vi "Lab Panel V6.00.vi"() -> ()   [LabVIEW 2017] (continued)
                n2534 = case shown="True" w4583 {
                  tunnel: w4587 -> [_ w4592]
                  tunnel: w4586 -> [_ w4591]
                  tunnel: w4585 -> [_ w4589]
                  tunnel: w4584 -> [_ w4588]
                  frame False {
                  }
                  frame True {
                    n2535 = local read "DISP LAB04-1"() -> (w4593:T4)
                    n2536 = local read "SIG LAB04-1"() -> (w4594:T2)
                    n2537 = local read "ON L04-1"() -> (w4590:cluster{"amps":dbl, "volts":dbl, "pf":dbl})
                    n2538 = Unbundle(w4594) -> ("AMPS"=w4600:dbl, "VOLTS"=w4598:dbl, "PF"=w4597:dbl, "Tmp Live"=w4596:dbl, "Tmp Neut"=w4599:dbl)
                    n2539 = Unbundle(w4593) -> ("CYCLE"=w4595:dbl)  [unwired: 2 out]
                    n2540 = stacked-sequence {
                      tunnel: w4600 -> [w4604 w4623]
                      tunnel: w4599 -> [_ w4622]
                      tunnel: w4598 -> [w4603 w4621]
                      tunnel: w4597 -> [w4602 w4620]
                      tunnel: w4596 -> [_ w4619]
                      tunnel: w4595 -> [_ w4618]
                      tunnel: w4592 -> [_ w4617]
                      tunnel: w4591 -> [w4605 _]
                      tunnel: w4590 -> [w4601 w4615]
                      tunnel: w4589 -> [_ w4616]
                      tunnel: w4588 -> [_ w4611]
                      frame #0 {
                        n2541 = case shown="True" w4605 {
                          tunnel: w4604 -> [_ w4610]
                          tunnel: w4603 -> [_ w4609]
                          tunnel: w4602 -> [_ w4608]
                          tunnel: w4601 -> [_ w4606]
                          frame False {
                          }
                          frame True {
                            n2542 = Bundle(cluster=w4606, "amps"=w4610, "volts"=w4609, "pf"=w4608) -> (w4607:cluster{"amps":dbl, "volts":dbl, "pf":dbl})
                            n2543 = local write "ON L04-1"(w4607) -> ()
                          }
                        }
                      }
                      frame #1 {
                        n2544 = Unbundle(w4615) -> ("amps"=w4614:dbl, "volts"=w4613:dbl, "pf"=w4612:dbl)
                        n2545 = case shown="True" w4616 {
                          tunnel: w4623 -> [_ w4655]
                          tunnel: w4622 -> [_ w4662]
                          tunnel: w4621 -> [_ _]
                          tunnel: w4620 -> [_ _]
                          tunnel: w4619 -> [_ w4661]
                          tunnel: w4618 -> [_ w4660]
                          tunnel: w4617 -> [_ w4625]
                          tunnel: w4614 -> [_ w4657]
                          tunnel: w4613 -> [_ w4656]
                          tunnel: w4612 -> [_ w4654]
                          tunnel: w4611 -> [_ w4646]
                          frame False {
                          }
                          frame True {
                            n2546 = local read "TDMS LAB04-1"() -> (w4659:refnum<k34>)
                            n2547 = Build Array(w4656) -> (w4651:dbl[])
                            n2548 = Build Array(w4654) -> (w4650:dbl[])
                            n2549 = Build Array(w4661) -> (w4649:dbl[])
                            n2550 = Build Array(w4662) -> (w4648:dbl[])
                            n2551 = Build Array(w4657) -> (w4653:dbl[])
                            n2552 = Build Array(w4655) -> (w4652:dbl[])
                            n2553 = Build Array(w4660) -> (w4647:dbl[])
                            n2554 = Build Array("AMPS ON", "AMPS OFF", "VOLTS", "PF", "TEMP Live", "TEMP Neut", "CYCLE") -> (w4630:string[])
                            n2555 = Bundle By Name("Y"=w4653, "t0"=w4646) -> (w4645:waveform(dbl))  [unwired: 1 in]
                            n2556 = Bundle By Name("Y"=w4652, "t0"=w4646) -> (w4644:waveform(dbl))  [unwired: 1 in]
                            n2557 = Bundle By Name("Y"=w4651, "t0"=w4646) -> (w4643:waveform(dbl))  [unwired: 1 in]
                            n2558 = Bundle By Name("Y"=w4650, "t0"=w4646) -> (w4642:waveform(dbl))  [unwired: 1 in]
                            n2559 = Bundle By Name("Y"=w4649, "t0"=w4646) -> (w4641:waveform(dbl))  [unwired: 1 in]
                            n2560 = Bundle By Name("Y"=w4648, "t0"=w4646) -> (w4640:waveform(dbl))  [unwired: 1 in]
                            n2561 = Bundle By Name("Y"=w4647, "t0"=w4646) -> (w4639:waveform(dbl))  [unwired: 1 in]
                            n2562 = Build Array(w4645, w4644, w4643, w4642, w4641, w4640, w4639) -> (w4638:waveform(dbl)[])
                            n2563 = TDMS Write(0:w4659, 5:"TEST VALUES", 7:w4630, 9:w4638) -> (4:w4629:refnum<k34>, 6:w4628:string, 15:w4627:errorcluster)  [unwired: 2 in, 1 out]
                            n2564 = TDMS Write(0:w4629, 5:w4628, 7:"TIME", 9:w4625, 11:w4627) -> (15:w4624:errorcluster)  [unwired: 1 in, 3 out]
                            n2565 = local write "data file error"(w4624) -> ()
                          }
                        }
                      }
                    }
                  }
                }
              }
              frame #7 {
                n2566 = case shown="True" w4663 {
                  tunnel: w4667 -> [_ w4672]
                  tunnel: w4666 -> [_ w4671]
                  tunnel: w4665 -> [_ w4669]
                  tunnel: w4664 -> [_ w4668]
                  frame False {
                  }
                  frame True {
                    n2567 = local read "DISP LAB04-2"() -> (w4673:T4)
                    n2568 = local read "SIG LAB04-2"() -> (w4674:T2)
                    n2569 = local read "ON L04-2"() -> (w4670:cluster{"amps":dbl, "volts":dbl, "pf":dbl})
                    n2570 = Unbundle(w4674) -> ("AMPS"=w4680:dbl, "VOLTS"=w4678:dbl, "PF"=w4677:dbl, "Tmp Live"=w4676:dbl, "Tmp Neut"=w4679:dbl)
                    n2571 = Unbundle(w4673) -> ("CYCLE"=w4675:dbl)  [unwired: 2 out]
                    n2572 = stacked-sequence {
                      tunnel: w4680 -> [w4684 w4703]
                      tunnel: w4679 -> [_ w4702]
                      tunnel: w4678 -> [w4683 w4701]
                      tunnel: w4677 -> [w4682 w4700]
                      tunnel: w4676 -> [_ w4699]
                      tunnel: w4675 -> [_ w4698]
                      tunnel: w4672 -> [_ w4697]
                      tunnel: w4671 -> [w4685 _]
                      tunnel: w4670 -> [w4681 w4695]
                      tunnel: w4669 -> [_ w4696]
                      tunnel: w4668 -> [_ w4691]
                      frame #0 {
                        n2573 = case shown="True" w4685 {
                          tunnel: w4684 -> [_ w4690]
                          tunnel: w4683 -> [_ w4689]
                          tunnel: w4682 -> [_ w4688]
                          tunnel: w4681 -> [_ w4686]
                          frame False {
                          }
                          frame True {
                            n2574 = Bundle(cluster=w4686, "amps"=w4690, "volts"=w4689, "pf"=w4688) -> (w4687:cluster{"amps":dbl, "volts":dbl, "pf":dbl})
                            n2575 = local write "ON L04-2"(w4687) -> ()
                          }
                        }
                      }
                      frame #1 {
                        n2576 = Unbundle(w4695) -> ("amps"=w4694:dbl, "volts"=w4693:dbl, "pf"=w4692:dbl)
                        n2577 = case shown="True" w4696 {
                          tunnel: w4703 -> [_ w4735]
                          tunnel: w4702 -> [_ w4742]
                          tunnel: w4701 -> [_ _]
                          tunnel: w4700 -> [_ _]
                          tunnel: w4699 -> [_ w4741]
                          tunnel: w4698 -> [_ w4740]
                          tunnel: w4697 -> [_ w4705]
                          tunnel: w4694 -> [_ w4737]
                          tunnel: w4693 -> [_ w4736]
                          tunnel: w4692 -> [_ w4734]
                          tunnel: w4691 -> [_ w4726]
                          frame False {
                          }
                          frame True {
                            n2578 = local read "TDMS LAB04-2"() -> (w4739:refnum<k34>)
                            n2579 = Build Array(w4736) -> (w4731:dbl[])
                            n2580 = Build Array(w4734) -> (w4730:dbl[])
                            n2581 = Build Array(w4741) -> (w4729:dbl[])
                            n2582 = Build Array(w4742) -> (w4728:dbl[])
                            n2583 = Build Array(w4737) -> (w4733:dbl[])
                            n2584 = Build Array(w4735) -> (w4732:dbl[])
                            n2585 = Build Array(w4740) -> (w4727:dbl[])
                            n2586 = Build Array("AMPS ON", "AMPS OFF", "VOLTS", "PF", "TEMP Live", "TEMP Neut", "CYCLE") -> (w4710:string[])
                            n2587 = Bundle By Name("Y"=w4733, "t0"=w4726) -> (w4725:waveform(dbl))  [unwired: 1 in]
                            n2588 = Bundle By Name("Y"=w4732, "t0"=w4726) -> (w4724:waveform(dbl))  [unwired: 1 in]
                            n2589 = Bundle By Name("Y"=w4731, "t0"=w4726) -> (w4723:waveform(dbl))  [unwired: 1 in]
                            n2590 = Bundle By Name("Y"=w4730, "t0"=w4726) -> (w4722:waveform(dbl))  [unwired: 1 in]
                            n2591 = Bundle By Name("Y"=w4729, "t0"=w4726) -> (w4721:waveform(dbl))  [unwired: 1 in]
                            n2592 = Bundle By Name("Y"=w4728, "t0"=w4726) -> (w4720:waveform(dbl))  [unwired: 1 in]
                            n2593 = Bundle By Name("Y"=w4727, "t0"=w4726) -> (w4719:waveform(dbl))  [unwired: 1 in]
                            n2594 = Build Array(w4725, w4724, w4723, w4722, w4721, w4720, w4719) -> (w4718:waveform(dbl)[])
                            n2595 = TDMS Write(0:w4739, 5:"TEST VALUES", 7:w4710, 9:w4718) -> (4:w4709:refnum<k34>, 6:w4708:string, 15:w4707:errorcluster)  [unwired: 2 in, 1 out]
                            n2596 = TDMS Write(0:w4709, 5:w4708, 7:"TIME", 9:w4705, 11:w4707) -> (15:w4704:errorcluster)  [unwired: 1 in, 3 out]
                            n2597 = local write "data file error"(w4704) -> ()
                          }
                        }
                      }
                    }
                  }
                }
              }
              frame #8 {
                n2598 = case shown="True" w4743 {
                  tunnel: w4747 -> [_ w4752]
                  tunnel: w4746 -> [_ w4751]
                  tunnel: w4745 -> [_ w4749]
                  tunnel: w4744 -> [_ w4748]
                  frame False {
                  }
                  frame True {
                    n2599 = local read "DISP LAB05-1"() -> (w4753:T4)
                    n2600 = local read "SIG LAB05-1"() -> (w4754:T2)
                    n2601 = local read "ON L05-1"() -> (w4750:cluster{"amps":dbl, "volts":dbl, "pf":dbl})
                    n2602 = Unbundle(w4754) -> ("AMPS"=w4760:dbl, "VOLTS"=w4758:dbl, "PF"=w4757:dbl, "Tmp Live"=w4756:dbl, "Tmp Neut"=w4759:dbl)
                    n2603 = Unbundle(w4753) -> ("CYCLE"=w4755:dbl)  [unwired: 2 out]
                    n2604 = stacked-sequence {
                      tunnel: w4760 -> [w4764 w4783]
                      tunnel: w4759 -> [_ w4782]
                      tunnel: w4758 -> [w4763 w4781]
                      tunnel: w4757 -> [w4762 w4780]
                      tunnel: w4756 -> [_ w4779]
                      tunnel: w4755 -> [_ w4778]
                      tunnel: w4752 -> [_ w4777]
                      tunnel: w4751 -> [w4765 _]
                      tunnel: w4750 -> [w4761 w4775]
                      tunnel: w4749 -> [_ w4776]
                      tunnel: w4748 -> [_ w4771]
                      frame #0 {
                        n2605 = case shown="True" w4765 {
                          tunnel: w4764 -> [_ w4770]
                          tunnel: w4763 -> [_ w4769]
                          tunnel: w4762 -> [_ w4768]
                          tunnel: w4761 -> [_ w4766]
                          frame False {
                          }
                          frame True {
                            n2606 = Bundle(cluster=w4766, "amps"=w4770, "volts"=w4769, "pf"=w4768) -> (w4767:cluster{"amps":dbl, "volts":dbl, "pf":dbl})
                            n2607 = local write "ON L05-1"(w4767) -> ()
                          }
                        }
                      }
                      frame #1 {
                        n2608 = Unbundle(w4775) -> ("amps"=w4774:dbl, "volts"=w4773:dbl, "pf"=w4772:dbl)
                        n2609 = case shown="True" w4776 {
                          tunnel: w4783 -> [_ w4815]
                          tunnel: w4782 -> [_ w4822]
                          tunnel: w4781 -> [_ _]
                          tunnel: w4780 -> [_ _]
                          tunnel: w4779 -> [_ w4821]
                          tunnel: w4778 -> [_ w4820]
                          tunnel: w4777 -> [_ w4785]
                          tunnel: w4774 -> [_ w4817]
                          tunnel: w4773 -> [_ w4816]
                          tunnel: w4772 -> [_ w4814]
                          tunnel: w4771 -> [_ w4806]
                          frame False {
                          }
                          frame True {
                            n2610 = local read "TDMS LAB05-1"() -> (w4819:refnum<k34>)
                            n2611 = Build Array(w4816) -> (w4811:dbl[])
                            n2612 = Build Array(w4814) -> (w4810:dbl[])
                            n2613 = Build Array(w4821) -> (w4809:dbl[])
                            n2614 = Build Array(w4822) -> (w4808:dbl[])
                            n2615 = Build Array(w4817) -> (w4813:dbl[])
                            n2616 = Build Array(w4815) -> (w4812:dbl[])
                            n2617 = Build Array(w4820) -> (w4807:dbl[])
                            n2618 = Build Array("AMPS ON", "AMPS OFF", "VOLTS", "PF", "TEMP Live", "TEMP Neut", "CYCLE") -> (w4790:string[])
                            n2619 = Bundle By Name("Y"=w4813, "t0"=w4806) -> (w4805:waveform(dbl))  [unwired: 1 in]
                            n2620 = Bundle By Name("Y"=w4812, "t0"=w4806) -> (w4804:waveform(dbl))  [unwired: 1 in]
                            n2621 = Bundle By Name("Y"=w4811, "t0"=w4806) -> (w4803:waveform(dbl))  [unwired: 1 in]
                            n2622 = Bundle By Name("Y"=w4810, "t0"=w4806) -> (w4802:waveform(dbl))  [unwired: 1 in]
                            n2623 = Bundle By Name("Y"=w4809, "t0"=w4806) -> (w4801:waveform(dbl))  [unwired: 1 in]
                            n2624 = Bundle By Name("Y"=w4808, "t0"=w4806) -> (w4800:waveform(dbl))  [unwired: 1 in]
                            n2625 = Bundle By Name("Y"=w4807, "t0"=w4806) -> (w4799:waveform(dbl))  [unwired: 1 in]
                            n2626 = Build Array(w4805, w4804, w4803, w4802, w4801, w4800, w4799) -> (w4798:waveform(dbl)[])
                            n2627 = TDMS Write(0:w4819, 5:"TEST VALUES", 7:w4790, 9:w4798) -> (4:w4789:refnum<k34>, 6:w4788:string, 15:w4787:errorcluster)  [unwired: 2 in, 1 out]
                            n2628 = TDMS Write(0:w4789, 5:w4788, 7:"TIME", 9:w4785, 11:w4787) -> (15:w4784:errorcluster)  [unwired: 1 in, 3 out]
                            n2629 = local write "data file error"(w4784) -> ()
                          }
                        }
                      }
                    }
                  }
                }
              }
              frame #9 {
                n2630 = case shown="True" w4823 {
                  tunnel: w4827 -> [_ w4832]
                  tunnel: w4826 -> [_ w4831]
                  tunnel: w4825 -> [_ w4829]
                  tunnel: w4824 -> [_ w4828]
                  frame False {
                  }
                  frame True {
                    n2631 = local read "DISP LAB05-2"() -> (w4833:T4)
                    n2632 = local read "SIG LAB05-2"() -> (w4834:T2)
                    n2633 = local read "ON L05-2"() -> (w4830:cluster{"amps":dbl, "volts":dbl, "pf":dbl})
                    n2634 = Unbundle(w4834) -> ("AMPS"=w4840:dbl, "VOLTS"=w4838:dbl, "PF"=w4837:dbl, "Tmp Live"=w4836:dbl, "Tmp Neut"=w4839:dbl)
                    n2635 = Unbundle(w4833) -> ("CYCLE"=w4835:dbl)  [unwired: 2 out]
                    n2636 = stacked-sequence {
                      tunnel: w4840 -> [w4844 w4863]
                      tunnel: w4839 -> [_ w4862]
                      tunnel: w4838 -> [w4843 w4861]
                      tunnel: w4837 -> [w4842 w4860]
                      tunnel: w4836 -> [_ w4859]
                      tunnel: w4835 -> [_ w4858]
                      tunnel: w4832 -> [_ w4857]
                      tunnel: w4831 -> [w4845 _]
                      tunnel: w4830 -> [w4841 w4855]
                      tunnel: w4829 -> [_ w4856]
                      tunnel: w4828 -> [_ w4851]
                      frame #0 {
                        n2637 = case shown="True" w4845 {
                          tunnel: w4844 -> [_ w4850]
                          tunnel: w4843 -> [_ w4849]
                          tunnel: w4842 -> [_ w4848]
                          tunnel: w4841 -> [_ w4846]
                          frame False {
                          }
                          frame True {
                            n2638 = Bundle(cluster=w4846, "amps"=w4850, "volts"=w4849, "pf"=w4848) -> (w4847:cluster{"amps":dbl, "volts":dbl, "pf":dbl})
                            n2639 = local write "ON L05-2"(w4847) -> ()
                          }
                        }
                      }
                      frame #1 {
                        n2640 = Unbundle(w4855) -> ("amps"=w4854:dbl, "volts"=w4853:dbl, "pf"=w4852:dbl)
                        n2641 = case shown="True" w4856 {
                          tunnel: w4863 -> [_ w4895]
                          tunnel: w4862 -> [_ w4902]
                          tunnel: w4861 -> [_ _]
                          tunnel: w4860 -> [_ _]
                          tunnel: w4859 -> [_ w4901]
                          tunnel: w4858 -> [_ w4900]
                          tunnel: w4857 -> [_ w4865]
                          tunnel: w4854 -> [_ w4897]
                          tunnel: w4853 -> [_ w4896]
                          tunnel: w4852 -> [_ w4894]
                          tunnel: w4851 -> [_ w4886]
                          frame False {
                          }
                          frame True {
                            n2642 = local read "TDMS LAB05-2"() -> (w4899:refnum<k34>)
                            n2643 = Build Array(w4896) -> (w4891:dbl[])
                            n2644 = Build Array(w4894) -> (w4890:dbl[])
                            n2645 = Build Array(w4901) -> (w4889:dbl[])
                            n2646 = Build Array(w4902) -> (w4888:dbl[])
                            n2647 = Build Array(w4897) -> (w4893:dbl[])
                            n2648 = Build Array(w4895) -> (w4892:dbl[])
                            n2649 = Build Array(w4900) -> (w4887:dbl[])
                            n2650 = Build Array("AMPS ON", "AMPS OFF", "VOLTS", "PF", "TEMP Live", "TEMP Neut", "CYCLE") -> (w4870:string[])
                            n2651 = Bundle By Name("Y"=w4893, "t0"=w4886) -> (w4885:waveform(dbl))  [unwired: 1 in]
                            n2652 = Bundle By Name("Y"=w4892, "t0"=w4886) -> (w4884:waveform(dbl))  [unwired: 1 in]
                            n2653 = Bundle By Name("Y"=w4891, "t0"=w4886) -> (w4883:waveform(dbl))  [unwired: 1 in]
                            n2654 = Bundle By Name("Y"=w4890, "t0"=w4886) -> (w4882:waveform(dbl))  [unwired: 1 in]
                            n2655 = Bundle By Name("Y"=w4889, "t0"=w4886) -> (w4881:waveform(dbl))  [unwired: 1 in]
                            n2656 = Bundle By Name("Y"=w4888, "t0"=w4886) -> (w4880:waveform(dbl))  [unwired: 1 in]
                            n2657 = Bundle By Name("Y"=w4887, "t0"=w4886) -> (w4879:waveform(dbl))  [unwired: 1 in]
                            n2658 = Build Array(w4885, w4884, w4883, w4882, w4881, w4880, w4879) -> (w4878:waveform(dbl)[])
                            n2659 = TDMS Write(0:w4899, 5:"TEST VALUES", 7:w4870, 9:w4878) -> (4:w4869:refnum<k34>, 6:w4868:string, 15:w4867:errorcluster)  [unwired: 2 in, 1 out]
                            n2660 = TDMS Write(0:w4869, 5:w4868, 7:"TIME", 9:w4865, 11:w4867) -> (15:w4864:errorcluster)  [unwired: 1 in, 3 out]
                            n2661 = local write "data file error"(w4864) -> ()
                          }
                        }
                      }
                    }
                  }
                }
              }
            }
          }
          frame #15 {
            # "display test values on chart"
            n2662 = local read "jig cycle"() -> (w4907:dbl)
            n2663 = local read "on loops"() -> (w4909:dbl)
            n2664 = Add(x=w4909, y=4) -> (x+y=w4906:dbl)
            n2665 = Equal?(x=w4907, y=3) -> (x = y?=w4905:bool)
            n2666 = Equal?(x=w4907, y=w4906) -> (x = y?=w4904:bool)
            n2667 = Or(x=w4905, y=w4904) -> (x .or. y?=w4903:bool)
            "graph flag" <- w4903
            n2668 = global write "Global display 3.vi" "graph flag"(w4903) -> ()
            n2669 = case shown="True" w4903 {
              frame False {
              }
              frame True {
                n2670 = local read "SIG LAB05-1"() -> (w4952:T2)
                n2671 = local read "SIG LAB04-2"() -> (w4953:T2)
                n2672 = local read "SIG LAB05-2"() -> (w4951:T2)
                n2673 = local read "SIG LAB04-1"() -> (w4954:T2)
                n2674 = local read "SIG LAB01-1"() -> (w4960:T2)
                n2675 = local read "SIG LAB03-1"() -> (w4956:T2)
                n2676 = local read "SIG LAB03-2"() -> (w4955:T2)
                n2677 = local read "SIG LAB02-2"() -> (w4957:T2)
                n2678 = local read "SIG LAB02-1"() -> (w4958:T2)
                n2679 = local read "SIG LAB01-2"() -> (w4959:T2)
                n2680 = Unbundle By Name(w4960) -> ("AMPS"=w4950:dbl, "VOLTS"=w4940:dbl, "Tmp Live"=w4930:dbl, "Tmp Neut"=w4920:dbl)
                n2681 = Unbundle(w4953) -> ("AMPS"=w4943:dbl, "VOLTS"=w4933:dbl, "Tmp Live"=w4923:dbl, "Tmp Neut"=w4913:dbl)  [unwired: 1 out]
                n2682 = Unbundle(w4952) -> ("AMPS"=w4942:dbl, "VOLTS"=w4932:dbl, "Tmp Live"=w4922:dbl, "Tmp Neut"=w4912:dbl)  [unwired: 1 out]
                n2683 = Unbundle(w4951) -> ("AMPS"=w4941:dbl, "VOLTS"=w4931:dbl, "Tmp Live"=w4921:dbl, "Tmp Neut"=w4911:dbl)  [unwired: 1 out]
                n2684 = Unbundle(w4954) -> ("AMPS"=w4944:dbl, "VOLTS"=w4934:dbl, "Tmp Live"=w4924:dbl, "Tmp Neut"=w4914:dbl)  [unwired: 1 out]
                n2685 = Unbundle(w4955) -> ("AMPS"=w4945:dbl, "VOLTS"=w4935:dbl, "Tmp Live"=w4925:dbl, "Tmp Neut"=w4915:dbl)  [unwired: 1 out]
                n2686 = Unbundle(w4956) -> ("AMPS"=w4946:dbl, "VOLTS"=w4936:dbl, "Tmp Live"=w4926:dbl, "Tmp Neut"=w4916:dbl)  [unwired: 1 out]
                n2687 = Unbundle(w4957) -> ("AMPS"=w4947:dbl, "VOLTS"=w4937:dbl, "Tmp Live"=w4927:dbl, "Tmp Neut"=w4917:dbl)  [unwired: 1 out]
                n2688 = Unbundle(w4958) -> ("AMPS"=w4948:dbl, "VOLTS"=w4938:dbl, "Tmp Live"=w4928:dbl, "Tmp Neut"=w4918:dbl)  [unwired: 1 out]
                n2689 = Unbundle(w4959) -> ("AMPS"=w4949:dbl, "VOLTS"=w4939:dbl, "Tmp Live"=w4929:dbl, "Tmp Neut"=w4919:dbl)  [unwired: 1 out]
                n2690 = stacked-sequence {
                  tunnel: w4950 -> [w4992 _ _]
                  tunnel: w4949 -> [w4991 _ _]
                  tunnel: w4948 -> [w4982 _ _]
                  tunnel: w4947 -> [w4981 _ _]
                  tunnel: w4946 -> [w4971 _ _]
                  tunnel: w4945 -> [w4970 _ _]
                  tunnel: w4944 -> [_ w5015 _]
                  tunnel: w4943 -> [_ w5014 _]
                  tunnel: w4942 -> [_ w5004 _]
                  tunnel: w4941 -> [_ w5003 _]
                  tunnel: w4940 -> [w4989 _ _]
                  tunnel: w4939 -> [w4988 _ _]
                  tunnel: w4938 -> [w4979 _ _]
                  tunnel: w4937 -> [w4978 _ _]
                  tunnel: w4936 -> [w4969 _ _]
                  tunnel: w4935 -> [w4968 _ _]
                  tunnel: w4934 -> [_ w5013 _]
                  tunnel: w4933 -> [_ w5012 _]
                  tunnel: w4932 -> [_ w5002 _]
                  tunnel: w4931 -> [_ w5001 _]
                  tunnel: w4930 -> [w4986 _ _]
                  tunnel: w4929 -> [w4984 _ _]
                  tunnel: w4928 -> [w4975 _ _]
                  tunnel: w4927 -> [w4973 _ _]
                  tunnel: w4926 -> [w4967 _ _]
                  tunnel: w4925 -> [w4965 _ _]
                  tunnel: w4924 -> [_ w5011 _]
                  tunnel: w4923 -> [_ w5009 _]
                  tunnel: w4922 -> [_ w5000 _]
                  tunnel: w4921 -> [_ w4998 _]
                  tunnel: w4920 -> [w4985 _ _]
                  tunnel: w4919 -> [w4983 _ _]
                  tunnel: w4918 -> [w4974 _ _]
                  tunnel: w4917 -> [w4972 _ _]
                  tunnel: w4916 -> [w4966 _ _]
                  tunnel: w4915 -> [w4964 _ _]
                  tunnel: w4914 -> [_ w5010 _]
                  tunnel: w4913 -> [_ w5008 _]
                  tunnel: w4912 -> [_ w4999 _]
                  tunnel: w4911 -> [_ w4997 _]
                  frame #0 {
                    n2691 = Merge Signals(w4992, w4991) -> (→"LAB01 AMPS":dynamicdata)
                    n2692 = Merge Signals(w4989, w4988) -> (→"LAB01 VOLTS":dynamicdata)
                    n2693 = Merge Signals(w4969, w4968) -> (→"LAB03 VOLTS":dynamicdata)
                    n2694 = Merge Signals(w4986, w4985, w4984, w4983) -> (→"LAB01 deg C":dynamicdata)
                    n2695 = Merge Signals(w4982, w4981) -> (→"LAB02 AMPS":dynamicdata)
                    n2696 = Merge Signals(w4975, w4974, w4973, w4972) -> (→"LAB02 deg C":dynamicdata)
                    n2697 = Merge Signals(w4967, w4966, w4965, w4964) -> (→"LAB03 deg C":dynamicdata)
                    n2698 = Merge Signals(w4979, w4978) -> (→"LAB02 VOLTS":dynamicdata)
                    n2699 = Merge Signals(w4971, w4970) -> (→"LAB03 AMPS":dynamicdata)
                  }
                  frame #1 {
                    n2700 = Merge Signals(w5002, w5001) -> (→"LAB05 VOLTS":dynamicdata)
                    n2701 = Merge Signals(w5015, w5014) -> (→"LAB04 AMPS":dynamicdata)
                    n2702 = Merge Signals(w5004, w5003) -> (→"LAB05 AMPS":dynamicdata)
                    n2703 = Merge Signals(w5000, w4999, w4998, w4997) -> (→"LAB05 deg C":dynamicdata)
                    n2704 = Merge Signals(w5011, w5010, w5009, w5008) -> (→"LAB04 deg C":dynamicdata)
                    n2705 = Merge Signals(w5013, w5012) -> (→"LAB04 VOLTS":dynamicdata)
                  }
                  frame #2 {
                    n2706 = local read "LAB05 VOLTS"() -> (w5023:dynamicdata)
                    n2707 = local read "LAB04 VOLTS"() -> (w5024:dynamicdata)
                    n2708 = local read "LAB05 AMPS"() -> (w5029:dynamicdata)
                    n2709 = local read "LAB02 VOLTS"() -> (w5026:dynamicdata)
                    n2710 = local read "LAB03 VOLTS"() -> (w5025:dynamicdata)
                    n2711 = local read "LAB01 VOLTS"() -> (w5027:dynamicdata)
                    n2712 = local read "LAB04 AMPS"() -> (w5030:dynamicdata)
                    n2713 = local read "LAB03 AMPS"() -> (w5031:dynamicdata)
                    n2714 = local read "LAB03 deg C"() -> (w5019:dynamicdata)
                    n2715 = local read "LAB02 AMPS"() -> (w5032:dynamicdata)
                    n2716 = local read "LAB04 deg C"() -> (w5018:dynamicdata)
                    n2717 = local read "LAB05 deg C"() -> (w5017:dynamicdata)
                    n2718 = local read "LAB02 deg C"() -> (w5020:dynamicdata)
                    n2719 = local read "LAB01 deg C"() -> (w5021:dynamicdata)
                    n2720 = local read "LAB01 AMPS"() -> (w5033:dynamicdata)
                    n2721 = Merge Signals(w5021, w5020, w5019, w5018, w5017) -> (w5016:dynamicdata)
                    n2722 = Merge Signals(w5033, w5032, w5031, w5030, w5029) -> (w5028:dynamicdata)
                    n2723 = Merge Signals(w5027, w5026, w5025, w5024, w5023) -> (w5022:dynamicdata)
                    n2724 = global write "Global display 3.vi" "graph volts"(w5022) -> ()
                    n2725 = global write "Global display 3.vi" "graph deg C"(w5016) -> ()
                    n2726 = global write "Global display 3.vi" "graph amps"(w5028) -> ()
                  }
                }
              }
            }
          }
          frame #16 {
            # "check for amps fail"
            # "check for cycle test & temperature rise fail conditions"
            n2727 = local read "on loops"() -> (w5061:dbl)
            n2728 = local read "jig cycle"() -> (w5058:dbl)
            n2729 = Add(x=w5061, y=5.0) -> (x+y=w5059:dbl)
            n2730 = Equal?(x=w5058, y=w5059) -> (x = y?=w5054:bool)
            n2731 = local read "jig cycle"() -> (w5063:dbl)
            n2732 = local read "TempErrors"() -> (w5034:bool[])
            n2733 = Equal?(x=w5063, y=3.0) -> (x = y?=w5056:bool)
            n2734 = local read "Fail Loops"() -> (w5035:dbl)
            n2735 = stacked-sequence {
              tunnel: w5057 -> [w5070 _ _ _ _ _ _ _ _ _]
              tunnel: w5056 -> [w5071 w5096 w5122 w5148 w5174 w5200 w5226 w5252 w5278 w5304]
              tunnel: w5055 -> [w5067 _ _ _ _ _ _ _ _ _]
              tunnel: w5054 -> [w5069 w5095 w5121 w5147 w5173 w5199 w5225 w5251 w5277 w5303]
              tunnel: w5053 -> [_ w5093 _ _ _ _ _ _ _ _]
              tunnel: w5052 -> [_ w5094 _ _ _ _ _ _ _ _]
              tunnel: w5051 -> [_ _ w5116 _ _ _ _ _ _ _]
              tunnel: w5050 -> [_ _ w5120 _ _ _ _ _ _ _]
              tunnel: w5049 -> [_ _ _ w5143 _ _ _ _ _ _]
              tunnel: w5048 -> [_ _ _ w5146 _ _ _ _ _ _]
              tunnel: w5047 -> [_ _ _ _ w5167 _ _ _ _ _]
              tunnel: w5046 -> [_ _ _ _ w5172 _ _ _ _ _]
              tunnel: w5045 -> [_ _ _ _ _ w5193 _ _ _ _]
              tunnel: w5044 -> [_ _ _ _ _ w5198 _ _ _ _]
              tunnel: w5043 -> [_ _ _ _ _ _ w5219 _ _ _]
              tunnel: w5042 -> [_ _ _ _ _ _ w5224 _ _ _]
              tunnel: w5041 -> [_ _ _ _ _ _ _ w5245 _ _]
              tunnel: w5040 -> [_ _ _ _ _ _ _ w5250 _ _]
              tunnel: w5039 -> [_ _ _ _ _ _ _ _ w5271 _]
              tunnel: w5038 -> [_ _ _ _ _ _ _ _ w5276 _]
              tunnel: w5037 -> [_ _ _ _ _ _ _ _ _ w5297]
              tunnel: w5036 -> [_ _ _ _ _ _ _ _ _ w5302]
              tunnel: w5034 -> [w5068 w5091 w5118 w5140 w5168 w5194 w5220 w5246 w5272 w5298]
              frame #0 {
                # "LAB01-1"
                n2736 = Index Array(array=w5068) -> (element=w5066:bool)  [unwired: 1 in]
                n2737 = Not(x=w5066) -> (.not. x?=w5065:bool)
                n2738 = And(x=w5065, y=w5067) -> (x .and. y?=w5064:bool)
                n2739 = case shown="True" w5064 {
                  tunnel: w5071 -> [_ w5085]
                  tunnel: w5070 -> [_ w5082]
                  tunnel: w5069 -> [_ w5081]
                  frame False {
                  }
                  frame True {
                    n2740 = local read "TEMP START LAB01-1"() -> (w5087:cluster{"TL":dbl, "TN":dbl})
                    n2741 = local read "RESULT LAB01-1"() -> (w5076:bool)
                    n2742 = local read "FAIL LAB01-1"() -> (w5079:cluster{"LO":dbl, "HI":dbl})
                    n2743 = local read "TDMS LAB01-1"() -> (w5086:refnum<k34>)
                    n2744 = local read "SET LAB01-1"() -> (w5083:T6)
                    n2745 = local read "DISP LAB01-1"() -> (w5084:T4)
                    n2746 = local read "SIG LAB01-1"() -> (w5088:T2)
                    n2747 = Bundle("FAIL LAB01-1"=w5079, "SIG LAB01-1"=w5088, "TEMP START LAB01-1"=w5087, "DISP LAB01-1"=w5084, "SET LAB01-1"=w5083, "TDMS LAB01-1"=w5086) -> (w5073:T37)  [unwired: 1 in]
                    n2748 = call "sub vi - cycle&temp fail v7.vi"("Amps Lo?"=w5085, "Input Cluster"=w5073, "SELECT"=w5082, "Amps Hi?"=w5081, "Result In"=w5076, "Panel"=u64 1) -> ("(FAIL) out"=w5078:cluster{"FAIL LO":dbl, "FAIL HI":dbl}, "(DISP) out"=w5074:T4, "T-RISE"=w5075:cluster{"T-RISE (L)":dbl, "T-RISE (N)":dbl}, "Result Out"=w5077:bool, "file error"=w5080:errorcluster)  [unwired: 9 in]
                    n2749 = local write "TEMP RISE LAB01-1"(w5075) -> ()
                    n2750 = local write "FAIL LAB01-1"(w5078) -> ()
                    n2751 = local write "DISP LAB01-1"(w5074) -> ()
                    n2752 = local write "RESULT LAB01-1"(w5077) -> ()
                    n2753 = local write "data file error"(w5080) -> ()
                  }
                }
              }
              frame #1 {
                # "LAB01-2"
                n2754 = Index Array(array=w5091) -> (element=w5092:bool)  [unwired: 1 in]
                n2755 = Not(x=w5092) -> (.not. x?=w5090:bool)
                n2756 = And(x=w5090, y=w5093) -> (x .and. y?=w5089:bool)
                n2757 = case shown="True" w5089 {
                  tunnel: w5096 -> [_ w5110]
                  tunnel: w5094 -> [_ w5107]
                  tunnel: w5095 -> [_ w5106]
                  frame False {
                  }
                  frame True {
                    n2758 = local read "TEMP START LAB01-2"() -> (w5112:cluster{"TL":dbl, "TN":dbl})
                    n2759 = local read "TDMS LAB01-2"() -> (w5111:refnum<k34>)
                    n2760 = local read "SET LAB01-2"() -> (w5108:T5)
                    n2761 = local read "DISP LAB01-2"() -> (w5109:T4)
                    n2762 = local read "FAIL LAB01-2"() -> (w5103:cluster{"LO":dbl, "HI":dbl})
                    n2763 = local read "RESULT LAB01-2"() -> (w5100:bool)
                    n2764 = local read "SIG LAB01-2"() -> (w5113:T2)
                    n2765 = Bundle("FAIL LAB01-2"=w5103, "SIG LAB01-2"=w5113, "TEMP START LAB01-2"=w5112, "DISP LAB01-2"=w5109, "SET LAB01-2"=w5108, "TDMS LAB01-2"=w5111) -> (w5098:T38)  [unwired: 1 in]
                    n2766 = call "sub vi - cycle&temp fail v7.vi"("Amps Lo?"=w5110, "Input Cluster"=w5098, "SELECT"=w5107, "Amps Hi?"=w5106, "Result In"=w5100, "Panel"=u64 2) -> ("(FAIL) out"=w5102:cluster{"FAIL LO":dbl, "FAIL HI":dbl}, "(DISP) out"=w5105:T4, "T-RISE"=w5099:cluster{"T-RISE (L)":dbl, "T-RISE (N)":dbl}, "Result Out"=w5101:bool, "file error"=w5104:errorcluster)  [unwired: 9 in]
                    n2767 = local write "TEMP RISE LAB01-2"(w5099) -> ()
                    n2768 = local write "FAIL LAB01-2"(w5102) -> ()
                    n2769 = local write "DISP LAB01-2"(w5105) -> ()
                    n2770 = local write "RESULT LAB01-2"(w5101) -> ()
                    n2771 = local write "data file error"(w5104) -> ()
                  }
                }
              }
              frame #2 {
                # "LAB02-1"
                n2772 = Index Array(array=w5118, index=1) -> (element=w5119:bool)
                n2773 = Not(x=w5119) -> (.not. x?=w5115:bool)
                n2774 = And(x=w5115, y=w5116) -> (x .and. y?=w5114:bool)
                n2775 = case shown="True" w5114 {
                  tunnel: w5122 -> [_ w5136]
                  tunnel: w5120 -> [_ w5133]
                  tunnel: w5121 -> [_ w5132]
                  frame False {
                  }
                  frame True {
                    n2776 = local read "TEMP START LAB02-1"() -> (w5138:cluster{"TL":dbl, "TN":dbl})
                    n2777 = local read "FAIL LAB02-1"() -> (w5129:cluster{"LO":dbl, "HI":dbl})
                    n2778 = local read "TDMS LAB02-1"() -> (w5137:refnum<k34>)
                    n2779 = local read "SIG LAB02-1"() -> (w5139:T2)
                    n2780 = local read "DISP LAB02-1"() -> (w5135:T4)
                    n2781 = local read "SET LAB02-1"() -> (w5134:T5)
                    n2782 = local read "RESULT LAB02-1"() -> (w5126:bool)
                    n2783 = Bundle("FAIL LAB02-1"=w5129, "SIG LAB02-1"=w5139, "TEMP START LAB02-1"=w5138, "DISP LAB02-1"=w5135, "SET LAB02-1"=w5134, "TDMS LAB02-1"=w5137) -> (w5124:T39)  [unwired: 1 in]
                    n2784 = call "sub vi - cycle&temp fail v7.vi"("Amps Lo?"=w5136, "Input Cluster"=w5124, "SELECT"=w5133, "Amps Hi?"=w5132, "Result In"=w5126, "Panel"=u64 3) -> ("(FAIL) out"=w5128:cluster{"FAIL LO":dbl, "FAIL HI":dbl}, "(DISP) out"=w5131:T4, "T-RISE"=w5125:cluster{"T-RISE (L)":dbl, "T-RISE (N)":dbl}, "Result Out"=w5127:bool, "file error"=w5130:errorcluster)  [unwired: 9 in]
                    n2785 = local write "DISP LAB02-1"(w5131) -> ()
                    n2786 = local write "data file error"(w5130) -> ()
                    n2787 = local write "TEMP RISE LAB02-1"(w5125) -> ()
                    n2788 = local write "RESULT LAB02-1"(w5127) -> ()
                    n2789 = local write "FAIL LAB02-1"(w5128) -> ()
                  }
                }
              }
              frame #3 {
                # "LAB02-2"
                n2790 = Index Array(array=w5140, index=1) -> (element=w5142:bool)
                n2791 = Not(x=w5142) -> (.not. x?=w5144:bool)
                n2792 = And(x=w5144, y=w5143) -> (x .and. y?=w5141:bool)
                n2793 = case shown="True" w5141 {
                  tunnel: w5148 -> [_ w5162]
                  tunnel: w5146 -> [_ w5159]
                  tunnel: w5147 -> [_ w5158]
                  frame False {
                  }
                  frame True {
                    n2794 = local read "TEMP START LAB02-2"() -> (w5164:cluster{"TL":dbl, "TN":dbl})
                    n2795 = local read "FAIL LAB02-2"() -> (w5155:cluster{"LO":dbl, "HI":dbl})
                    n2796 = local read "TDMS LAB02-2"() -> (w5163:refnum<k34>)
                    n2797 = local read "SET LAB02-2"() -> (w5160:T5)
                    n2798 = local read "DISP LAB02-2"() -> (w5161:T4)
                    n2799 = local read "SIG LAB02-2"() -> (w5165:T2)
                    n2800 = local read "RESULT LAB02-2"() -> (w5152:bool)
                    n2801 = Bundle("FAIL LAB02-2"=w5155, "SIG LAB02-2"=w5165, "TEMP START LAB02-2"=w5164, "DISP LAB02-2"=w5161, "SET LAB02-2"=w5160, "TDMS LAB02-2"=w5163) -> (w5150:T40)  [unwired: 1 in]
                    n2802 = call "sub vi - cycle&temp fail v7.vi"("Amps Lo?"=w5162, "Input Cluster"=w5150, "SELECT"=w5159, "Amps Hi?"=w5158, "Result In"=w5152, "Panel"=u64 4) -> ("(FAIL) out"=w5154:cluster{"FAIL LO":dbl, "FAIL HI":dbl}, "(DISP) out"=w5157:T4, "T-RISE"=w5151:cluster{"T-RISE (L)":dbl, "T-RISE (N)":dbl}, "Result Out"=w5153:bool, "file error"=w5156:errorcluster)  [unwired: 9 in]
                    n2803 = local write "TEMP RISE LAB02-2"(w5151) -> ()
                    n2804 = local write "FAIL LAB02-2"(w5154) -> ()
                    n2805 = local write "DISP LAB02-2"(w5157) -> ()
                    n2806 = local write "RESULT LAB02-2"(w5153) -> ()
                    n2807 = local write "data file error"(w5156) -> ()
                  }
                }
              }
              frame #4 {
                # "LAB03-1"
                n2808 = Index Array(array=w5168, index=2) -> (element=w5171:bool)
                n2809 = Not(x=w5171) -> (.not. x?=w5169:bool)
                n2810 = And(x=w5169, y=w5167) -> (x .and. y?=w5166:bool)
                n2811 = case shown="True" w5166 {
                  tunnel: w5174 -> [_ w5188]
                  tunnel: w5172 -> [_ w5185]
                  tunnel: w5173 -> [_ w5184]
                  frame False {
                  }
                  frame True {
                    n2812 = local read "TEMP START LAB03-1"() -> (w5190:cluster{"TL":dbl, "TN":dbl})
                    n2813 = local read "FAIL LAB03-1"() -> (w5181:cluster{"LO":dbl, "HI":dbl})
                    n2814 = local read "TDMS LAB03-1"() -> (w5189:refnum<k34>)
                    n2815 = local read "SET LAB03-1"() -> (w5186:T5)
                    n2816 = local read "DISP LAB03-1"() -> (w5187:T4)
                    n2817 = local read "SIG LAB03-1"() -> (w5191:T2)
                    n2818 = local read "RESULT LAB03-1"() -> (w5178:bool)
                    n2819 = Bundle("FAIL LAB03-1"=w5181, "SIG LAB03-1"=w5191, "TEMP START LAB03-1"=w5190, "DISP LAB03-1"=w5187, "SET LAB03-1"=w5186, "TDMS LAB03-1"=w5189) -> (w5176:T41)  [unwired: 1 in]
                    n2820 = call "sub vi - cycle&temp fail v7.vi"("Amps Lo?"=w5188, "Input Cluster"=w5176, "SELECT"=w5185, "Amps Hi?"=w5184, "Result In"=w5178, "Panel"=u64 5) -> ("(FAIL) out"=w5180:cluster{"FAIL LO":dbl, "FAIL HI":dbl}, "(DISP) out"=w5183:T4, "T-RISE"=w5177:cluster{"T-RISE (L)":dbl, "T-RISE (N)":dbl}, "Result Out"=w5179:bool, "file error"=w5182:errorcluster)  [unwired: 9 in]
                    n2821 = local write "TEMP RISE LAB03-1"(w5177) -> ()
                    n2822 = local write "FAIL LAB03-1"(w5180) -> ()
                    n2823 = local write "DISP LAB03-1"(w5183) -> ()
                    n2824 = local write "RESULT LAB03-1"(w5179) -> ()
                    n2825 = local write "data file error"(w5182) -> ()
                  }
                }
              }
              frame #5 {
                # "LAB03-2"
                n2826 = Index Array(array=w5194, index=2) -> (element=w5197:bool)
                n2827 = Not(x=w5197) -> (.not. x?=w5195:bool)
                n2828 = And(x=w5195, y=w5193) -> (x .and. y?=w5192:bool)
                n2829 = case shown="True" w5192 {
                  tunnel: w5200 -> [_ w5214]
                  tunnel: w5198 -> [_ w5211]
                  tunnel: w5199 -> [_ w5210]
                  frame False {
                  }
                  frame True {
                    n2830 = local read "TEMP START LAB03-2"() -> (w5216:cluster{"TL":dbl, "TN":dbl})
                    n2831 = local read "FAIL LAB03-2"() -> (w5207:cluster{"LO":dbl, "HI":dbl})
                    n2832 = local read "TDMS LAB03-2"() -> (w5215:refnum<k34>)
                    n2833 = local read "SET LAB03-2"() -> (w5212:T5)
                    n2834 = local read "DISP LAB03-2"() -> (w5213:T4)
                    n2835 = local read "RESULT LAB03-2"() -> (w5204:bool)
                    n2836 = local read "SIG LAB03-2"() -> (w5217:T2)
                    n2837 = Bundle("FAIL LAB03-2"=w5207, "SIG LAB03-2"=w5217, "TEMP START LAB03-2"=w5216, "DISP LAB03-2"=w5213, "SET LAB03-2"=w5212, "TDMS LAB03-2"=w5215) -> (w5202:T42)  [unwired: 1 in]
                    n2838 = call "sub vi - cycle&temp fail v7.vi"("Amps Lo?"=w5214, "Input Cluster"=w5202, "SELECT"=w5211, "Amps Hi?"=w5210, "Result In"=w5204, "Panel"=u64 6) -> ("(FAIL) out"=w5206:cluster{"FAIL LO":dbl, "FAIL HI":dbl}, "(DISP) out"=w5209:T4, "T-RISE"=w5203:cluster{"T-RISE (L)":dbl, "T-RISE (N)":dbl}, "Result Out"=w5205:bool, "file error"=w5208:errorcluster)  [unwired: 9 in]
                    n2839 = local write "FAIL LAB03-2"(w5206) -> ()
                    n2840 = local write "TEMP RISE LAB03-2"(w5203) -> ()
                    n2841 = local write "DISP LAB03-2"(w5209) -> ()
                    n2842 = local write "RESULT LAB03-2"(w5205) -> ()
                    n2843 = local write "data file error"(w5208) -> ()
                  }
                }
              }
              frame #6 {
                # "LAB04-1"
                n2844 = Index Array(array=w5220, index=3) -> (element=w5223:bool)
                n2845 = Not(x=w5223) -> (.not. x?=w5221:bool)
                n2846 = And(x=w5221, y=w5219) -> (x .and. y?=w5218:bool)
                n2847 = case shown="True" w5218 {
                  tunnel: w5226 -> [_ w5240]
                  tunnel: w5224 -> [_ w5237]
                  tunnel: w5225 -> [_ w5236]
                  frame False {
                  }
                  frame True {
                    n2848 = local read "TEMP START LAB04-1"() -> (w5242:cluster{"TL":dbl, "TN":dbl})
                    n2849 = local read "FAIL LAB04-1"() -> (w5233:cluster{"LO":dbl, "HI":dbl})
                    n2850 = local read "TDMS LAB04-1"() -> (w5241:refnum<k34>)
                    n2851 = local read "SET LAB04-1"() -> (w5238:T5)
                    n2852 = local read "DISP LAB04-1"() -> (w5239:T4)
                    n2853 = local read "SIG LAB04-1"() -> (w5243:T2)
                    n2854 = local read "RESULT LAB04-1"() -> (w5230:bool)
                    n2855 = Bundle("FAIL LAB04-1"=w5233, "SIG LAB04-1"=w5243, "TEMP START LAB04-1"=w5242, "DISP LAB04-1"=w5239, "SET LAB04-1"=w5238, "TDMS LAB04-1"=w5241) -> (w5228:T43)  [unwired: 1 in]
                    n2856 = call "sub vi - cycle&temp fail v7.vi"("Amps Lo?"=w5240, "Input Cluster"=w5228, "SELECT"=w5237, "Amps Hi?"=w5236, "Result In"=w5230, "Panel"=u64 7) -> ("(FAIL) out"=w5232:cluster{"FAIL LO":dbl, "FAIL HI":dbl}, "(DISP) out"=w5235:T4, "T-RISE"=w5229:cluster{"T-RISE (L)":dbl, "T-RISE (N)":dbl}, "Result Out"=w5231:bool, "file error"=w5234:errorcluster)  [unwired: 9 in]
                    n2857 = local write "TEMP RISE LAB04-1"(w5229) -> ()
                    n2858 = local write "FAIL LAB04-1"(w5232) -> ()
                    n2859 = local write "DISP LAB04-1"(w5235) -> ()
                    n2860 = local write "RESULT LAB04-1"(w5231) -> ()
                    n2861 = local write "data file error"(w5234) -> ()
                  }
                }
              }
              frame #7 {
                # "LAB04-2"
                n2862 = Index Array(array=w5246, index=3) -> (element=w5249:bool)
                n2863 = Not(x=w5249) -> (.not. x?=w5247:bool)
                n2864 = And(x=w5247, y=w5245) -> (x .and. y?=w5244:bool)
                n2865 = case shown="True" w5244 {
                  tunnel: w5252 -> [_ w5266]
                  tunnel: w5250 -> [_ w5263]
                  tunnel: w5251 -> [_ w5262]
                  frame False {
                  }
                  frame True {
                    n2866 = local read "TEMP START LAB04-2"() -> (w5268:cluster{"TL":dbl, "TN":dbl})
                    n2867 = local read "FAIL LAB04-2"() -> (w5259:cluster{"LO":dbl, "HI":dbl})
                    n2868 = local read "TDMS LAB04-2"() -> (w5267:refnum<k34>)
                    n2869 = local read "SET LAB04-2"() -> (w5264:T5)
                    n2870 = local read "DISP LAB04-2"() -> (w5265:T4)
                    n2871 = local read "SIG LAB04-2"() -> (w5269:T2)
                    n2872 = local read "RESULT LAB04-2"() -> (w5256:bool)
                    n2873 = Bundle("FAIL LAB04-2"=w5259, "SIG LAB04-2"=w5269, "TEMP START LAB04-2"=w5268, "DISP LAB04-2"=w5265, "SET LAB04-2"=w5264, "TDMS LAB04-2"=w5267) -> (w5254:T44)  [unwired: 1 in]
                    n2874 = call "sub vi - cycle&temp fail v7.vi"("Amps Lo?"=w5266, "Input Cluster"=w5254, "SELECT"=w5263, "Amps Hi?"=w5262, "Result In"=w5256, "Panel"=u64 8) -> ("(FAIL) out"=w5258:cluster{"FAIL LO":dbl, "FAIL HI":dbl}, "(DISP) out"=w5261:T4, "T-RISE"=w5255:cluster{"T-RISE (L)":dbl, "T-RISE (N)":dbl}, "Result Out"=w5257:bool, "file error"=w5260:errorcluster)  [unwired: 9 in]
                    n2875 = local write "TEMP RISE LAB04-2"(w5255) -> ()
                    n2876 = local write "FAIL LAB04-2"(w5258) -> ()
                    n2877 = local write "DISP LAB04-2"(w5261) -> ()
                    n2878 = local write "RESULT LAB04-2"(w5257) -> ()
                    n2879 = local write "data file error"(w5260) -> ()
                  }
                }
              }
              frame #8 {
                # "LAB05-1"
                n2880 = Index Array(array=w5272, index=4) -> (element=w5275:bool)
                n2881 = Not(x=w5275) -> (.not. x?=w5273:bool)
                n2882 = And(x=w5273, y=w5271) -> (x .and. y?=w5270:bool)
                n2883 = case shown="True" w5270 {
                  tunnel: w5278 -> [_ w5292]
                  tunnel: w5276 -> [_ w5289]
                  tunnel: w5277 -> [_ w5288]
                  frame False {
                  }
                  frame True {
                    n2884 = local read "TEMP START LAB05-1"() -> (w5294:cluster{"TL":dbl, "TN":dbl})
                    n2885 = local read "FAIL LAB05-1"() -> (w5285:cluster{"LO":dbl, "HI":dbl})
                    n2886 = local read "TDMS LAB05-1"() -> (w5293:refnum<k34>)
                    n2887 = local read "SET LAB05-1"() -> (w5290:T5)
                    n2888 = local read "DISP LAB05-1"() -> (w5291:T4)
                    n2889 = local read "SIG LAB05-1"() -> (w5295:T2)
                    n2890 = local read "RESULT LAB05-1"() -> (w5282:bool)
                    n2891 = Bundle("FAIL LAB05-1"=w5285, "SIG LAB05-1"=w5295, "TEMP START LAB05-1"=w5294, "DISP LAB05-1"=w5291, "SET LAB05-1"=w5290, "TDMS LAB05-1"=w5293) -> (w5280:T45)  [unwired: 1 in]
                    n2892 = call "sub vi - cycle&temp fail v7.vi"("Amps Lo?"=w5292, "Input Cluster"=w5280, "SELECT"=w5289, "Amps Hi?"=w5288, "Result In"=w5282, "Panel"=u64 9) -> ("(FAIL) out"=w5284:cluster{"FAIL LO":dbl, "FAIL HI":dbl}, "(DISP) out"=w5287:T4, "T-RISE"=w5281:cluster{"T-RISE (L)":dbl, "T-RISE (N)":dbl}, "Result Out"=w5283:bool, "file error"=w5286:errorcluster)  [unwired: 9 in]
                    n2893 = local write "TEMP RISE LAB05-1"(w5281) -> ()
                    n2894 = local write "FAIL LAB05-1"(w5284) -> ()
                    n2895 = local write "DISP LAB05-1"(w5287) -> ()
                    n2896 = local write "RESULT LAB05-1"(w5283) -> ()
                    n2897 = local write "data file error"(w5286) -> ()
                  }
                }
              }
              frame #9 {
                # "LAB05-2"
